vi "SPC_get_sync_state.vi"(8 "Error In":errorcluster, 10 "Module No":i16 min=0 max=7 step=1, 11 "DLL Path":path) -> (0 "Error Out":errorcluster, 1 "SYNC State Value":i16, 2 "Module No":i16, 3 "DLL Path":path, 4 "Sync Status":bool)   [LabVIEW 2023]
doc: "The procedure sets \"sync_state\" according to the actual sync state on the SPC module ‘mod_no’.\n\nFor SPC-130(140)(930) module possible values are:\n0: SYNC NOT OK, sync input not triggered\n1: SYNC OK, sync input triggers\n\nFor other SPC modules possible values are:\n0: NO SYNC, sync input not triggered\n1: SYNC OK, sync input triggers\n2, 3: SYNC OVERLOAD.\n\ninfo@becker-hickl.com"
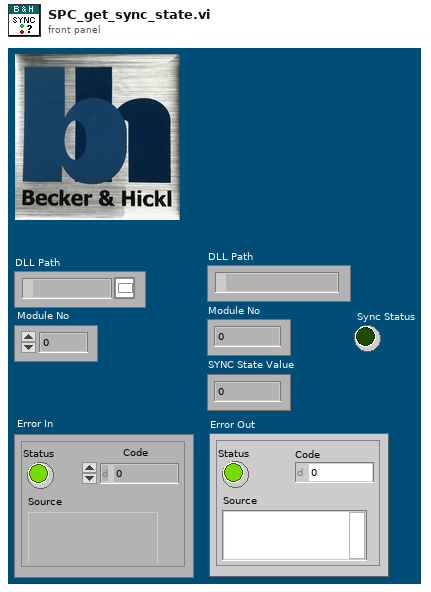
[diagram p1: front panel]
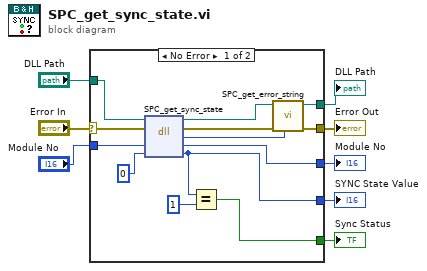
[diagram p0: block diagram]
diagram:
  n1 = case shown="No Error" "Error In" {
    selector: "Error In" -> [w20 w24]
    tunnel: "DLL Path" -> [w21 w23]
    tunnel: [w11 w24] -> w6
    tunnel: [w15 w23] -> w5
    tunnel: [w13 _] -> w4
    tunnel: [w14 w22] -> w3
    tunnel: "Module No" -> [w19 w22]
    tunnel: [w10 _] -> w1
    frame No Error {
      n2 = dll-call lib="D:/spcm/lib/lab_view/lv10.0/spcm32.dll" fn="SPC_get_sync_state"(path in=w21, error in=w20, "mod_no"=w19, "sync_state"=i16 0 ("Sync State")) -> (path out=w16:path, error out=w17:errorcluster, "return type"=w18:i16, "mod_no"=w14:i16, "sync_state"=w13:i16)  [unwired: 1 in]
      n3 = Equal?(x=w13, y=i16 1) -> (x = y?=w10:bool)
      n4 = call "SPC_get_error_string.vi"("ErrorID"=w18, "Error In"=w17, "DLL Path"=w16) -> ("Error Out"=w11:errorcluster, "DLL Path"=w15:path)  [unwired: 6 in, 1 out]
    }
    frame Error {
    }
  }
  "DLL Path" <- w5
  "Error Out" <- w6
  "SYNC State Value" <- w4
  "Module No" <- w3
  "Sync Status" <- w1
